vi "Write CFG File.vi"(8 "error in (no error)":errorcluster, 10 "File path":path, 11 "Mag Lab Root in":refnum<class "Mag Lab Root.lvclass">) -> (0 "error out":errorcluster, 3 "Mag Lab Root out":refnum<class "Mag Lab Root.lvclass">)   [LabVIEW 2015, in "Mag Lab Root.lvclass"]
uses:
  Mag Lab Root.lvclass
  Mag Lab Root.lvclass/Mag Lab Root.ctl
  Mag Lab Properties/Mag Lab Parameters.lvclass
  <vilib>/Utility/config.llb/NI_LVConfig.lvlib
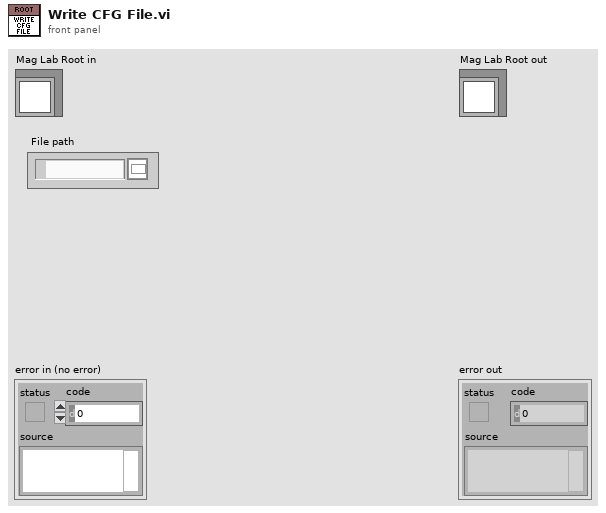
[diagram p1: front panel]
types:
  T1 = typedef "NI_LVConfig.lvlib/Config Data RefNum.ctl" = refnum<k1>
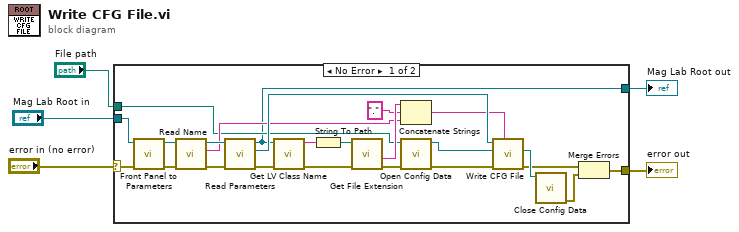
[diagram p0: block diagram]
diagram:
  n1 = case shown="No Error" "error in (no error)" {
    selector: "error in (no error)" -> [w19 w31]
    tunnel: [w15 w31] -> w4
    tunnel: [w10 w30] -> w2
    tunnel: "Mag Lab Root in" -> [w29 w30]
    tunnel: "File path" -> [w20 _]
    frame No Error {
      n2 = call-dynamic "Front Panel to Parameters.vi"("error in (no error)"=w19, "Mag Lab Root in"=w29) -> ("error out"=w26:errorcluster, "Mag Lab Root out"=w27:refnum<class "Mag Lab Root.lvclass">)  [unwired: 8 in]
      n3 = call "Read Name.vi"("error in (no error)"=w26, "Mag Lab Root in"=w27) -> ("error out"=w25:errorcluster, "Name"=w21:string, "Mag Lab Root out"=w28:refnum<class "Mag Lab Root.lvclass">)  [unwired: 7 in]
      n4 = call-dynamic "Read Parameters.vi"("error in (no error)"=w25, "Mag Lab Root in"=w28) -> ("error out"=w12:errorcluster, "Mag Lab Parameters.lvclass"=w24:refnum<class "Mag Lab Parameters.lvclass">, "Mag Lab Root out"=w10:refnum<class "Mag Lab Root.lvclass">)  [unwired: 7 in]
      n5 = call <vilib>:"Get LV Class Name.vi"("error in (no error)"=w12, "object"=w10) -> ("error out"=w11:errorcluster, "class name"=w8:string)  [unwired: 8 in]
      n6 = String To Path(string=w8) -> (path=w23:path)
      n7 = call <vilib>:"Get File Extension.vi"("error in (no error)"=w11, "file"=w23) -> ("error out"=w18:errorcluster, "filename without extension"=w22:string)  [unwired: 5 in, 3 out]
      n8 = Concatenate Strings(w22, "." ("string"), w21) -> (w9:string)
      n9 = call <vilib>:"Open Config Data.vi"("error in (no error)"=w18, "configuration file path"=w20) -> ("error out"=w6:errorcluster, "refnum"=w7:T1)  [unwired: 7 in, 1 out]
      n10 = call-dynamic "Write CFG File.vi"("Section"=w9, "error in (no error)"=w6, "File refnum"=w7, "Mag Lab Parameters in"=w24) -> ("error out"=w16:errorcluster, "File refnum out"=w17:T1)  [unwired: 5 in, 1 out]
      n11 = call <vilib>:"Close Config Data.vi"("refnum"=w17) -> ("error out"=w14:errorcluster)  [unwired: 9 in, 1 out]
      n12 = Merge Errors(w16, w14) -> (w15:errorcluster)
    }
    frame Error {
    }
  }
  "error out" <- w4
  "Mag Lab Root out" <- w2
